vi "TDMS Viewer.vi"   [LabVIEW 2016]
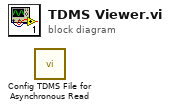
[diagram p0: block diagram]
diagram:
  n1 = call "Config TDMS File for Asynchronous Read.vi"() -> ()  [unwired: 13 in, 3 out]
